vi "MFLI set variable parameters.vi"(8 "error in":errorcluster, 10 "ACQ parameters":T2={"Filter order"=5.0, "Filter tau [ms]"=9.0, "F_Mod [kHz]"=1.0, "Amp_Mod [mV]"=0.0, "Enable output"=0, "Phase [°]"=0.0} {"Enable output" items=["Disable", "Enable"]; "Filter order" min=1.0 step=1.0; "Filter tau [ms]" min=1.0 max=9.0 step=1.0}, 11 "handle in":T1 {"Handle" format="0x%08x"; "Conn" format="0x%08x"}) -> (0 "Error Out":errorcluster, 3 "Handle Out":T1 {"Handle" format="0x%08x"; "Conn" format="0x%08x"})   [LabVIEW 2024, in "Lock-in module.lvlib"]
uses:
  Lock-in module.lvlib
  ctl/MFLI parameters.ctl
  <instrlib>/Zurich Instruments LabOne/Public/ziTypeHandle.ctl
  <instrlib>/Zurich Instruments LabOne/Public/Configure/ziSetValueDouble.vi
  <instrlib>/Zurich Instruments LabOne/Zurich Instruments LabOne.lvlib
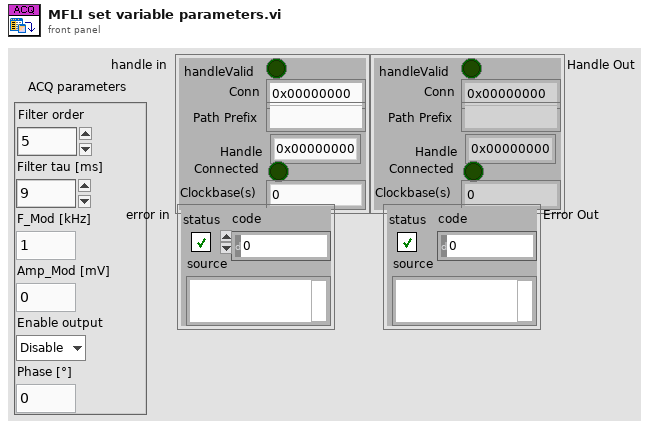
[diagram p1: front panel]
types:
  T1 = typedef "Zurich Instruments LabOne.lvlib/ziTypeHandle.ctl" = cluster{"handleValid":bool, "Conn":u64, "Path Prefix":string, "Handle":u64, "Connected":bool, "Clockbase(s)":dbl}
  T2 = typedef "Lock-in module.lvlib/MFLI parameters.ctl" = cluster{"Filter order":dbl, "Filter tau [ms]":dbl, "F_Mod [kHz]":dbl, "Amp_Mod [mV]":dbl, "Enable output":u16, "Phase [°]":dbl}
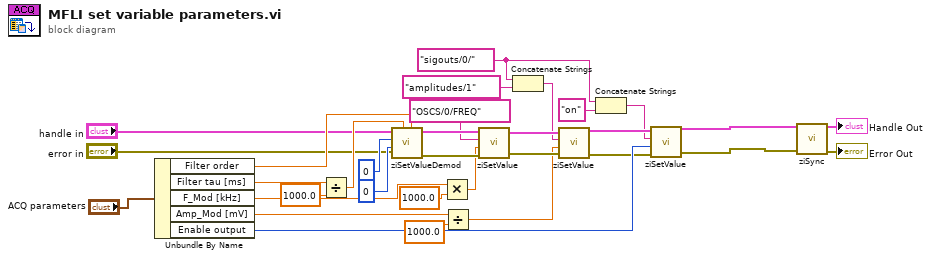
[diagram p0: block diagram]
diagram:
  w25 = "sigouts/0/" ("string")
  n1 = Unbundle By Name("ACQ parameters") -> ("Filter order"=w18:dbl, "Filter tau [ms]"=w19:dbl, "F_Mod [kHz]"=w11:dbl, "Amp_Mod [mV]"=w9:dbl, "Enable output"=w32:u16)
  n2 = Divide(x=w19, y=1000.0) -> (x/y=w15:dbl)
  n3 = call <instrlib>:"ziSetValueDemod.vi"("Order (2)"=w18, "Time Constant (1ms)"=w15, "error in"="error in", "Signal Input Select (0)"=0, "Demodulator # (0)"=0, "handle in"="handle in") -> ("error out"=w31:errorcluster, "handle out"=w30:T1)  [unwired: 4 in]
  n4 = Multiply(x=w11, y=1000.0) -> (x*y=w10:dbl)
  n5 = Divide(x=w9, y=1000.0) -> (x/y=w23:dbl)
  n6 = call-poly <instrlib>:"ziSetValue.vi"("Error In"=w31, "Value"=w10, "Path"="OSCS/0/FREQ", "Handle In"=w30) -> ("Error Out"=w29:errorcluster, "Handle Out"=w28:T1)  [unwired: 1 in]
  n7 = Concatenate Strings(w25, "amplitudes/1") -> (w22:string)
  n8 = call-poly <instrlib>:"ziSetValue.vi"("Error In"=w29, "Value"=w23, "Path"=w22, "Handle In"=w28) -> ("Error Out"=w27:errorcluster, "Handle Out"=w26:T1)  [unwired: 1 in]
  n9 = Concatenate Strings(w25, "on" ("Path")) -> (w21:string)
  n10 = call-poly <instrlib>:"ziSetValue.vi"("Error In"=w27, "Value"=w32, "Path"=w21, "Handle In"=w26) -> ("Error Out"=w1:errorcluster, "Handle Out"=w2:T1)  [unwired: 1 in]
  n11 = call <instrlib>:"ziSync.vi"("Handle In"=w2, "Error In"=w1) -> ("Handle Out"=→"Handle Out":T1, "Error Out"=→"Error Out":errorcluster)  [unwired: 12 in]
